vi "Comparision operators.vi"() -> ()   [LabVIEW 2019]
panel:
  out "x > y?":bool
  out "x <= y?":bool
  out "x >= y?":bool
  out "x < y?":bool
  out "x != y?":bool
  out "x = y?":bool
  in  "Y":dbl
  in  "X":dbl
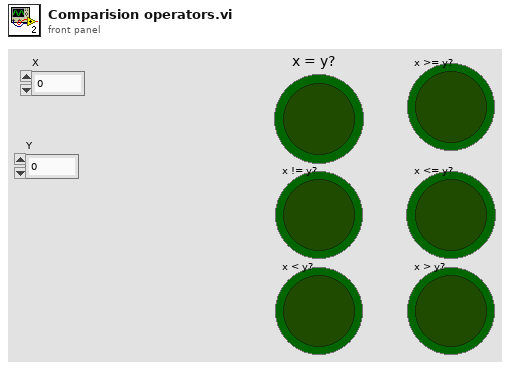
[diagram p1: front panel]
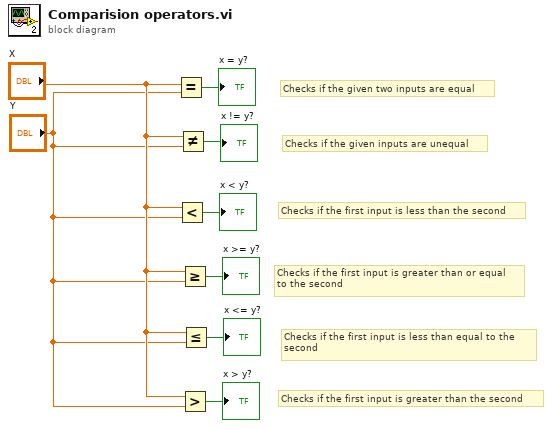
[diagram p0: block diagram]
diagram:
  # "Checks if the first input is greater than the second"
  # "Checks if the first input is less than equal to the \nsecond"
  # "Checks if the first input is greater than or equal\nto the second"
  # "Checks if the first input is less than the second"
  # "Checks if the given inputs are unequal"
  # "Checks if the given two inputs are equal"
  n1 = Equal?(x="X", y="Y") -> (x = y?=→"x = y?":bool)
  n2 = Less?(x="X", y="Y") -> (x < y?=→"x < y?":bool)
  n3 = Not Equal?(x="X", y="Y") -> (x != y?=→"x != y?":bool)
  n4 = Greater Or Equal?(x="X", y="Y") -> (x >= y?=→"x >= y?":bool)
  n5 = Greater?(x="X", y="Y") -> (0:→"x > y?":bool)
  n6 = Less Or Equal?(x="X", y="Y") -> (x <= y?=→"x <= y?":bool)
